vi "Memory.Pointer.Offset to Address (safe).vi"(8 "error in (no error)":errorcluster, 10 "offset":i64 format="%d bytes", 11 "Pointer in":refnum<class "Memory.Pointer.lvclass">) -> (0 "error out":errorcluster, 1 "valid address":bool, 2 "address":u64 format="%016x", 3 "Pointer out":refnum<class "Memory.Pointer.lvclass">)   [LabVIEW 2016, in "LabVIEW Memory Manager.lvlib" / "Memory.Pointer.lvclass"]
uses:
  Memory.Pointer.lvclass
  Memory.Pointer.lvclass/Memory.Pointer.ctl
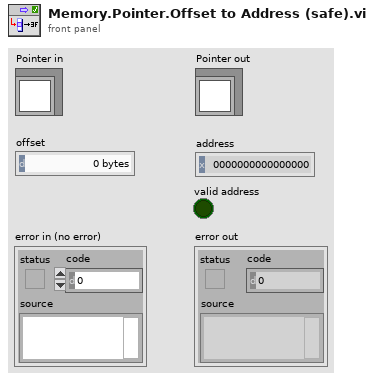
[diagram p1: front panel]
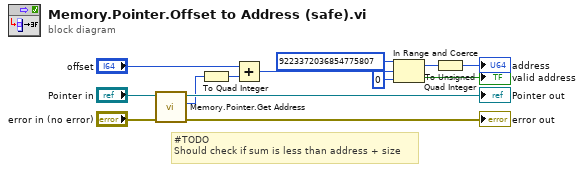
[diagram p0: block diagram]
diagram:
  # "#TODO\nShould check if sum is less than address + size"
  n1 = call "Memory.Pointer.Get Address.vi"("error in (no error)"="error in (no error)", "Pointer in"="Pointer in") -> ("error out"=→"error out":errorcluster, "address"=w8:u64, "Pointer out"=→"Pointer out":refnum<class "Memory.Pointer.lvclass">)  [unwired: 7 in]
  n2 = To Quad Integer(1:w8) -> (0:w7:i64)
  n3 = Add(x="offset", y=w7) -> (x+y=w5:i64)
  n4 = In Range and Coerce(upper limit=i64 9223372036854775807, x=w5, lower limit=i64 0) -> (coerced(x)=w2:i64, In Range?=→"valid address":bool)
  n5 = To Unsigned Quad Integer(1:w2) -> (0:→"address":u64)
